vi "Img Update Basic Point.vi"(8 "error in (no error)":errorcluster, 11 "LF2R IDE in":refnum<class "Main Panel.lvclass">) -> (0 "error out":errorcluster, 3 "LF2R IDE out":refnum<class "Main Panel.lvclass">)   [LabVIEW 2018, in "Main Panel.lvlib" / "Main Panel.lvclass"]
uses:
  Main Panel.lvclass
  Picture Process/Picture Process.lvclass
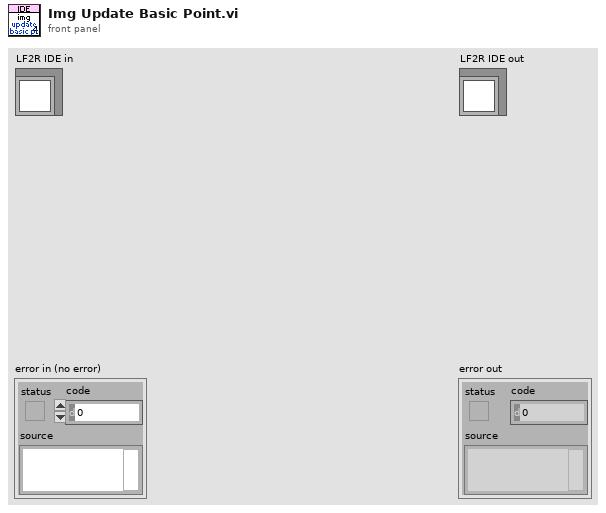
[diagram p1: front panel]
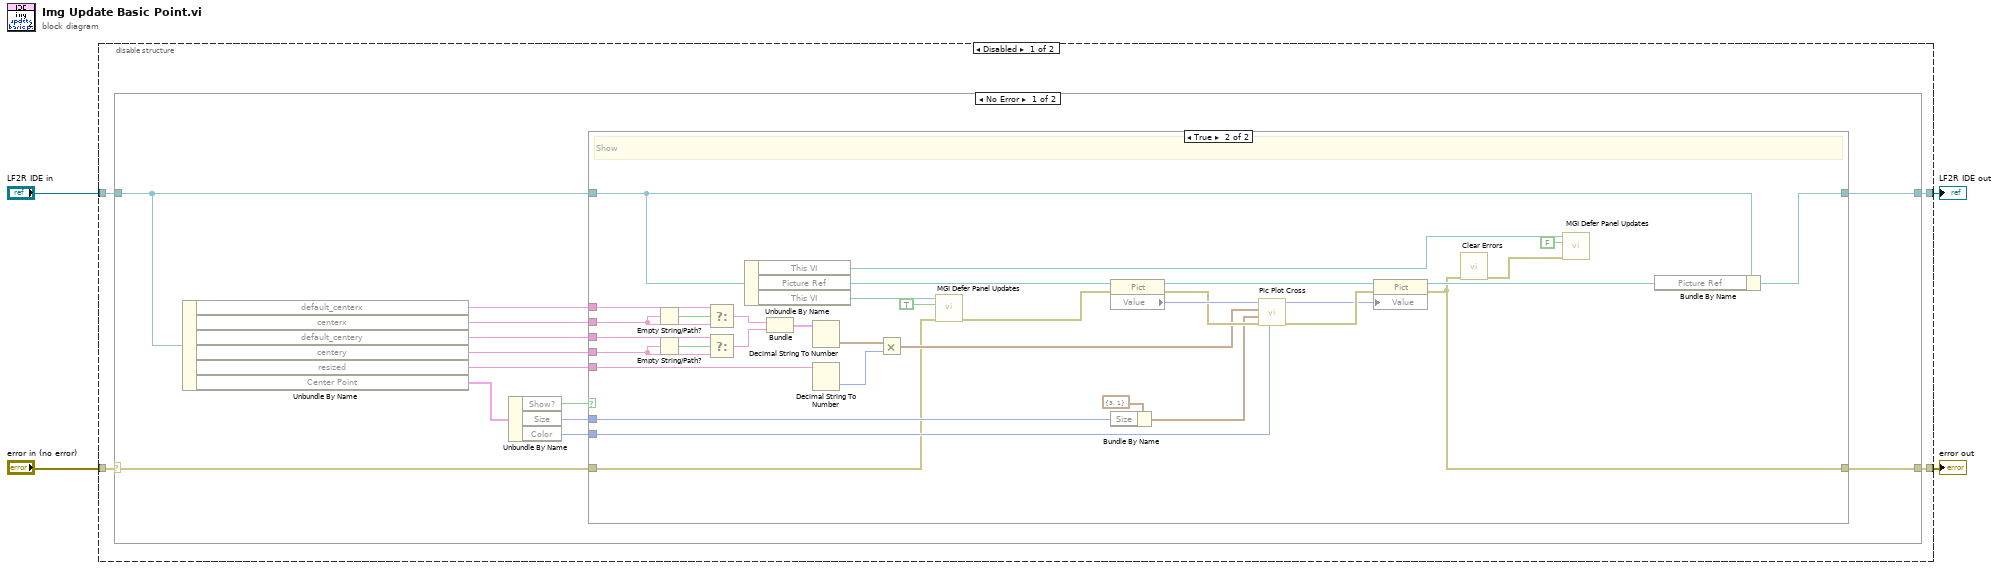
[diagram p0: block diagram]
diagram:
  n1 = disable-structure shown="Disabled" {
    disable-tunnel: "error in (no error)" -> [w8 w60]
    disable-tunnel: [w7 w60] -> w3
    disable-tunnel: "LF2R IDE in" -> [w6 w61]
    disable-tunnel: [w5 w61] -> w1
    frame Disabled {
      n2 = case shown="No Error" w8 {
        selector: w8 -> [w14 w59]
        tunnel: [w20 w59] -> w7
        tunnel: [w12 w58] -> w5
        tunnel: w6 -> [w21 w58]
        frame No Error {
          n3 = Unbundle By Name(w21) -> ("default_centerx"=w18:string, "centerx"=w17:string, "default_centery"=w16:string, "centery"=w15:string, "resized"=w19:string, "Center Point"=w13:cluster{"Size":i32, "Color":u32, "Show?":bool})
          n4 = Unbundle By Name(w13) -> ("Show?"=w11:bool, "Size"=w10:i32, "Color"=w9:u32)
          n5 = case shown="True" w11 {
            tunnel: w21 -> [w23 w45]
            tunnel: [w22 w28] -> w20
            tunnel: w19 -> [_ w57]
            tunnel: w18 -> [_ w53]
            tunnel: w17 -> [_ w52]
            tunnel: w16 -> [_ w50]
            tunnel: w15 -> [_ w49]
            tunnel: w14 -> [w22 w30]
            tunnel: [w23 w33] -> w12
            tunnel: w10 -> [_ w38]
            tunnel: w9 -> [_ w40]
            frame False {
              # "Skip"
            }
            frame True {
              # "Show"
              n6 = Empty String/Path?(string/path=w52) -> (empty?=w54:bool)
              n7 = Empty String/Path?(string/path=w49) -> (empty?=w51:bool)
              n8 = Select(t=w53, s=w54, f=w52) -> (s? t:f=w48:string)
              n9 = Select(t=w50, s=w51, f=w49) -> (s? t:f=w47:string)
              n10 = Unbundle By Name(w45) -> ("This VI"=w26:refnum<vi>, "Picture Ref"=w44:refnum<vi>, "This VI"=w31:refnum<vi>)
              n11 = Bundle("centerx"=w48, "centery"=w47) -> (w46:cluster{"centerx":string, "centery":string})  [unwired: 1 in]
              n12 = Decimal String To Number(string=w46) -> (number=w56:cluster{"centerx":i32, "centery":i32})  [unwired: 2 in, 1 out]
              n13 = Decimal String To Number(string=w57) -> (number=w55:i32)  [unwired: 2 in, 1 out]
              n14 = Multiply(x=w56, y=w55) -> (x*y=w41:cluster{"centerx":i32, "centery":i32})
              n15 = call <userlib>:"MGI Defer Panel Updates.vi"("Error In"=w30, "Defer Updates?"=TRUE, "VI Reference (Caller)"=w31) -> ("Error Out"=w29:errorcluster)  [unwired: 8 in]
              n16 = property class="Pict"(reference=w44, error in=w29) -> (reference out=w36:refnum<vi>, error out=w42:errorcluster, "Value"=w43:picture)
              n17 = Bundle By Name(cluster=cluster{"Size":i32, "Width":u16} {"Size"=3, "Width"=1} ("Line"), "Size"=w38) -> (w37:cluster{"Size":i32, "Width":u16})
              n18 = call "Pic Plot Cross.vi"("Color"=w40, "error in (no error)"=w42, "Line"=w37, "Position"=w41, "Picture in"=w43) -> ("error out"=w35:errorcluster, "Picture out"=w34:picture)  [unwired: 5 in]
              n19 = property class="Pict"(reference=w36, error in=w35, "Value"=w34) -> (reference out=w32:refnum<vi>, error out=w28:errorcluster)
              n20 = call <vilib>:"Clear Errors.vi"("error in (no error)"=w28) -> ("error out"=w27:errorcluster)  [unwired: 5 in, 1 out]
              n21 = call <userlib>:"MGI Defer Panel Updates.vi"("Error In"=w27, "Defer Updates?"=FALSE, "VI Reference (Caller)"=w26) -> ()  [unwired: 8 in, 1 out]
              n22 = Bundle By Name(cluster=w45, "Picture Ref"=w32) -> (w33:refnum<class "Main Panel.lvclass">)
            }
          }
        }
        frame Error {
        }
      }
    }
    frame Enabled {
    }
  }
  "error out" <- w3
  "LF2R IDE out" <- w1
